vi "Set Hint.vi"(8 "error in":errorcluster, 10 "Value":string="rb", 11 "Name":string(combo)) -> (0 "error out":errorcluster, 3 "Boolean":u32 format="%.0x")   [LabVIEW 2015, in "LibSDL2.lvlib"]
uses:
  LibSDL2.lvlib
  DLL/SDL2.dll
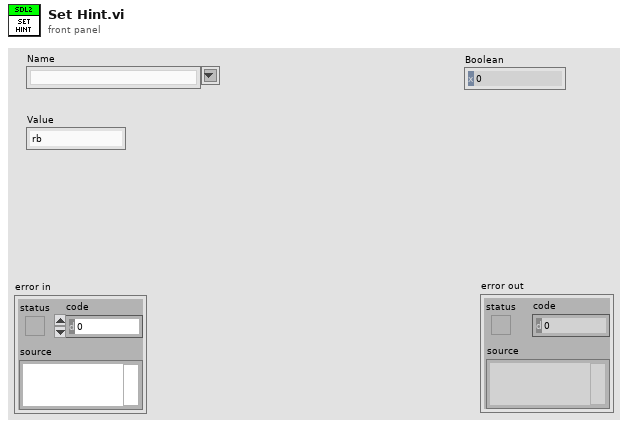
[diagram p1: front panel]
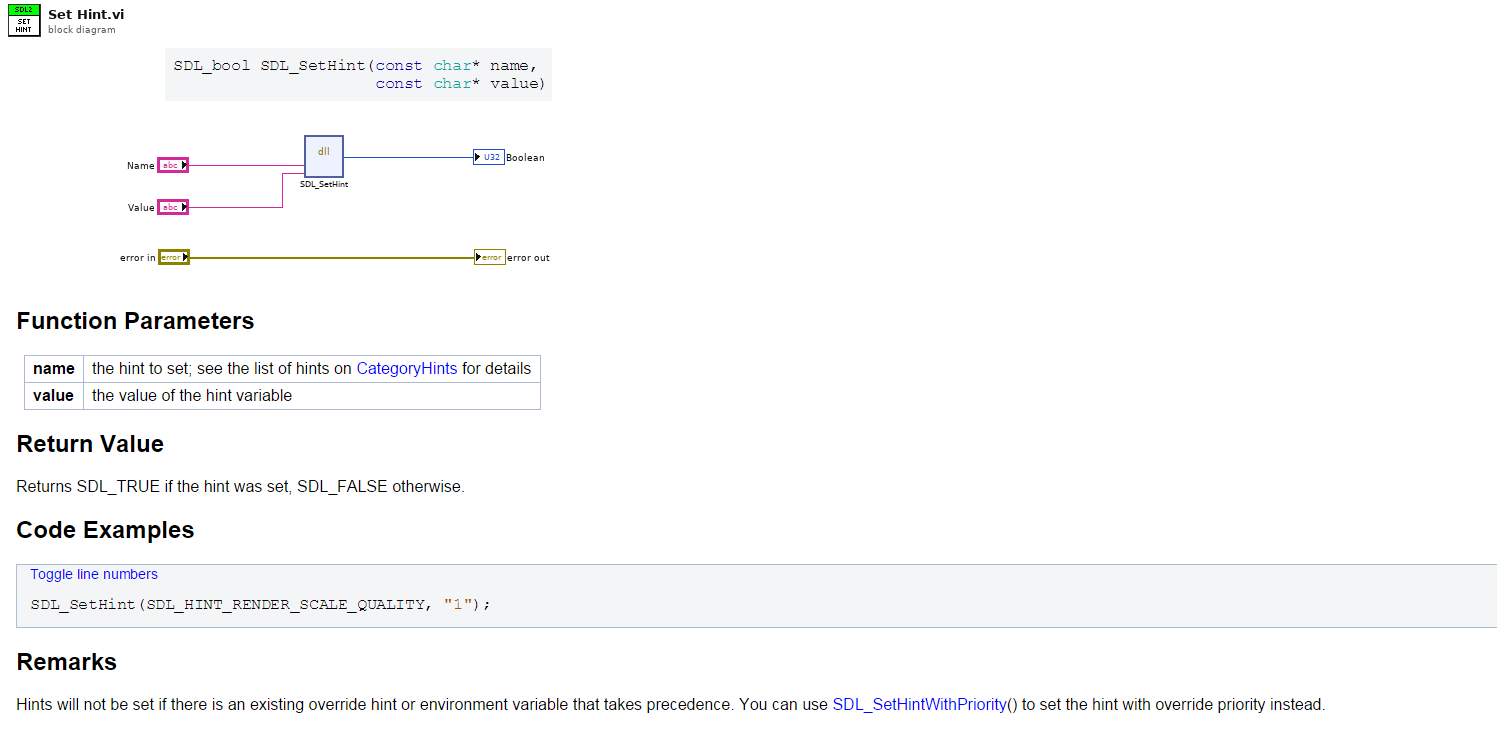
[diagram p0: block diagram]
diagram:
  n1 = dll-call lib="C:/dev/PGS/LabSDL2/Source/Libraries/LibSDL2 Wrapper/DLL/SDL2.dll" fn="SDL_SetHint"("name"="Name", "value"="Value") -> ("bool"=→"Boolean":u32)  [unwired: 5 in, 2 out]
  "error out" <- "error in"
